vi "BackupAndIntakeRTv2.vi"   [LabVIEW 2015]
uses:
  ShiftGlobals.vi
  MotorPositionGlobals.vi
  RobotCode/TwoBallAutoGlobals.vi
  GeneralGlobals.vi
types:
  T1 = typedef "WPI_MotorControlDeviceRef.ctl" = cluster{"DeviceStatus":errorcluster, "Type":T2, "PWM":cluster{"PWM Channel":T3, "DeadBand":T4}, "CAN":cluster{"Device Number":u8, "Control Mode":T5, "Semaphore":T6, "Max Vout":dbl, "TalonSRX Control Mode":T7}, "Invert":bool}
  T2 = typedef "WPI_MotorControlType.ctl" = enum16{"PWM", "CAN", "CANTalonSRX"}
  T3 = typedef "FPGA_DIOPWMChannel.ctl" = enum8{"PWM 0", "PWM 1", "PWM 2", "PWM 3", "PWM 4", "PWM 5", "PWM 6", "PWM 7", "PWM 8", "PWM 9", "PWM MXP 0", "PWM MXP 1", "PWM MXP 2", "PWM MXP 3", "PWM MXP 4", "PWM MXP 5", "PWM MXP 6", "PWM MXP 7", "PWM MXP 8", "PWM MXP 9", "Invalid"}
  T4 = typedef "WPI_PWMDeadband.ctl" = cluster{"Name":string, "maxPositivePwm":i32, "minPositivePwm":i32, "centerPwm":i32, "maxNegativePwm":i32, "minNegativePwm":i32, "angularRange":u16}
  T5 = typedef "WPI_CANJaguar_ControlMode.ctl" = enum8{"Percent VBus", "Current", "Speed", "Position", "Voltage"}
  T6 = typedef "Semaphore RefNum" = refnum<k1>
  T7 = typedef "WPI_CANTalonSRX_APIControlMode.ctl" = enum8{"Percent VBus", "Speed", "Position", "Slave", "Unchanged / Invalid", "Voltage Compensation", "Current", "Motion Profile"}
  T8 = typedef "WPI_CANTalonSRX_GlobalStatus.ctl" = cluster{"Applied Throttle":dbl, "Module Enabled":bool, "CAN Error":errorcluster, "Closed Loop Error":dbl, "Forward Limit Switch Closed":bool, "Reverse Limit Switch Closed":bool, "Sensor Position":dbl, "Sensor Velocity":dbl, "Current":dbl, "Sticky Fault - Over Temp":bool, "Sticky Fault - Under Voltage":bool, "Sticky Fault - Forward Limit":bool, "Sticky Fault - Reverse Limit":bool, "Sticky Fault - Forward Soft Limit":bool, "Sticky Fault - Reverse Soft Limit":bool, "Brake is Enabled":bool, "Encoder Position":dbl, "Encoder Velocity":dbl, "Encoder Index Count":dbl, "Encoder A Pin State":bool, "Encoder B Pin State":bool, "Encoder Index Pin State":bool, "Analog In":dbl, "Analog In Velocity":dbl, "Temperature (C)":dbl, "Battery Voltage":dbl, "Control 5 Is Supported":bool, "Current Profile Slot Select":dbl, "Pos Div 8":bool, "Vel Div 4":bool, "Pulse Width Position":i32, "Pulse Width Velocity":i32, "Pulse Width Rise To Rise (us)":i32, "Pulse Width Rise To Fall (us)":i32, "Mot Prof Active Is Under Run":bool, "Mot Prof Active Has Under Run":bool, "Mot Prof Active Is Last":bool, "Mot Prof Active Velocity Only":bool, "Mot Prof Active Is Valid":bool, "Mot Prof Buffer Is Full":bool, "Mot Prof Active Profile Slot Select":i32, "Mot Prof NextID":i32, "Mot Prof Count":i32, "Mot Prof Active Velocity":dbl, "Mot Prof Active Position":dbl, "Mot Prof Output Enable":i32}
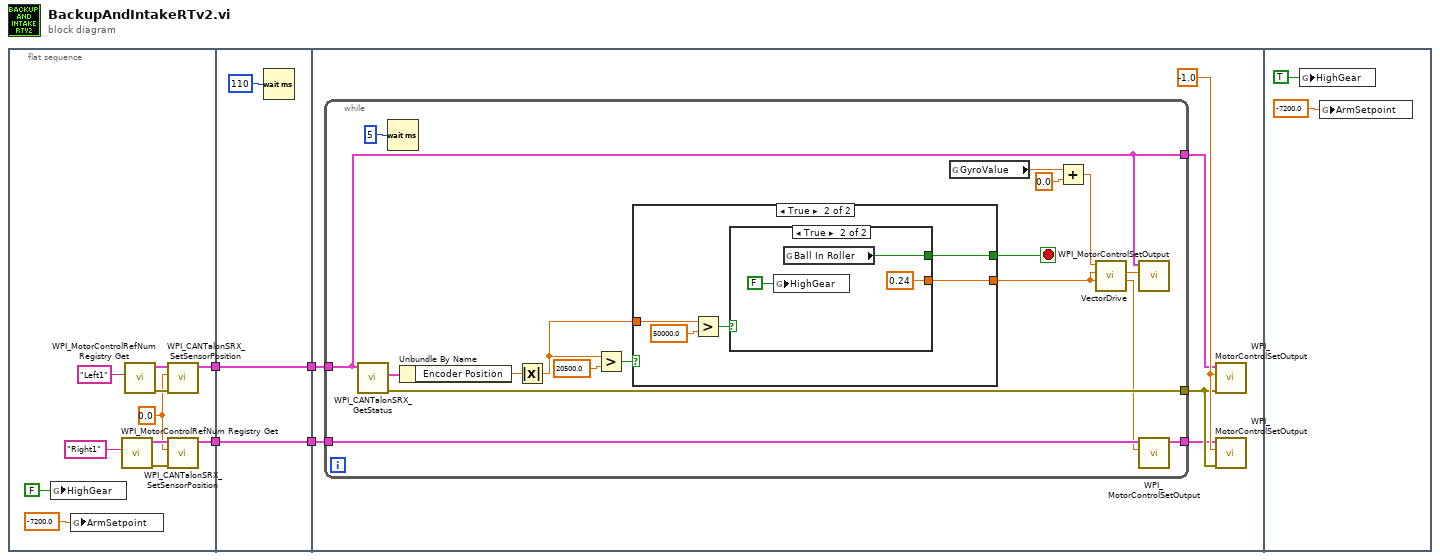
[diagram p0: block diagram]
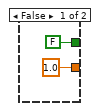
[diagram p2: hidden frame]
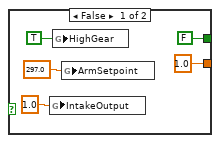
[diagram p3: hidden frame]
diagram:
  n1 = flat-sequence {
    tunnel: [w8] -> w4
    tunnel: [w7] -> w3
    tunnel: w4 -> [w18]
    tunnel: [w18] -> w1
    tunnel: w3 -> [w17]
    tunnel: [w17] -> w2
    tunnel: w2 -> [w22]
    tunnel: w1 -> [w21]
    frame #0 {
      w9 = 0.0 ("New Sensor Position")
      n2 = global write "ShiftGlobals.vi" "HighGear"(FALSE ("HighGear")) -> ()
      n3 = global write "MotorPositionGlobals.vi" "ArmSetpoint"(-7200.0 ("ArmSetpoint")) -> ()
      n4 = call <vilib>:"WPI_MotorControlRefNum Registry Get.vi"("refnum name"="Right1") -> ("error out"=w13:errorcluster, "MotorControlDevRef"=w12:T1)  [unwired: 9 in]
      n5 = call <vilib>:"WPI_MotorControlRefNum Registry Get.vi"("refnum name"="Left1") -> ("error out"=w11:errorcluster, "MotorControlDevRef"=w10:T1)  [unwired: 9 in]
      n6 = call <vilib>:"WPI_CANTalonSRX_SetSensorPosition.vi"("error in (no error)"=w11, "New Sensor Position"=w9, "CAN Talon SRX Ref"=w10) -> ("CAN Talon SRX Ref"=w7:T1)  [unwired: 7 in, 1 out]
      n7 = call <vilib>:"WPI_CANTalonSRX_SetSensorPosition.vi"("error in (no error)"=w13, "New Sensor Position"=w9, "CAN Talon SRX Ref"=w12) -> ("CAN Talon SRX Ref"=w8:T1)  [unwired: 7 in, 1 out]
    }
    frame #1 {
      n8 = Wait (ms)(milliseconds to wait=u32 110) -> ()  [unwired: 1 out]
    }
    frame #2 {
      w24 = -1.0 ("Output")
      n9 = while {
        tunnel: [w38] -> w23
        tunnel: w22 -> [w26]
        tunnel: w21 -> [w37]
        tunnel: [w26] -> w20
        tunnel: [w36] -> w19
        stop <- w25 stop-if-true
        n10 = call <vilib>:"WPI_CANTalonSRX_GetStatus.vi"("CAN Talon SRX Ref"=w26) -> ("error out"=w38:errorcluster, "Talon SRX Status"=w40:T8)  [unwired: 8 in, 1 out]
        n11 = Wait (ms)(milliseconds to wait=u32 5) -> ()  [unwired: 1 out]
        n12 = Unbundle By Name(w40) -> ("Encoder Position"=w39:dbl)
        n13 = Absolute Value(x=w39) -> (abs(x)=w28:dbl)
        n14 = Greater?(x=w28, y=20500.0) -> (0:w29:bool)
        n15 = case shown="True" w29 {
          tunnel: w28 -> [_ w47]
          tunnel: [1.0 ("Output") w45] -> w27
          tunnel: [FALSE ("HighGear") w44] -> w25
          frame False {
          }
          frame True {
            n16 = Greater?(x=w47, y=50000.0) -> (0:w48:bool)
            n17 = case shown="True" w48 {
              tunnel: [1.0 ("Output") 0.24 ("Output")] -> w45
              tunnel: [FALSE ("HighGear") w54] -> w44
              frame False {
                n18 = global write "MotorPositionGlobals.vi" "IntakeOutput"(1.0 ("IntakeOutput")) -> ()
                n19 = global write "ShiftGlobals.vi" "HighGear"(TRUE ("HighGear")) -> ()
                n20 = global write "MotorPositionGlobals.vi" "ArmSetpoint"(297.0 ("ArmSetpoint")) -> ()
              }
              frame True {
                n21 = global write "ShiftGlobals.vi" "HighGear"(FALSE ("HighGear")) -> ()
                n22 = global read "GeneralGlobals.vi" "Ball In Roller"() -> (w54:bool)
              }
            }
          }
        }
        n23 = global read "TwoBallAutoGlobals.vi" "GyroValue"() -> (w33:dbl)
        n24 = Add(x=w33, y=0.0 ("setpoint")) -> (x+y=w31:dbl)
        n25 = call "VectorDrive.vi"("RightMotorInput"=w27, "LeftMotorInput"=w27, "setpoint"=w31) -> ("RightMotorOutput"=w34:dbl, "LeftMotorOutput"=w35:dbl)  [unwired: 7 in]
        n26 = call <vilib>:"WPI_MotorControlSetOutput.vi"("Output"=w35, "MotorControlDevRef"=w26) -> ()  [unwired: 7 in, 3 out]
        n27 = call <vilib>:"WPI_MotorControlSetOutput.vi"("Output"=w34, "MotorControlDevRef"=w37) -> ("MotorControlDevRef"=w36:T1)  [unwired: 7 in, 2 out]
      }
      n28 = call <vilib>:"WPI_MotorControlSetOutput.vi"("error in (no error)"=w23, "Output"=w24, "MotorControlDevRef"=w20) -> ()  [unwired: 6 in, 3 out]
      n29 = call <vilib>:"WPI_MotorControlSetOutput.vi"("error in (no error)"=w23, "Output"=w24, "MotorControlDevRef"=w19) -> ()  [unwired: 6 in, 3 out]
    }
    frame #3 {
      n30 = global write "ShiftGlobals.vi" "HighGear"(TRUE ("HighGear")) -> ()
      n31 = global write "MotorPositionGlobals.vi" "ArmSetpoint"(-7200.0 ("ArmSetpoint")) -> ()
    }
  }
